vi "Configure Trigger.vi"(8 "error in (no error)":errorcluster, 10 "Params":variant, 11 "ConfigTrigger in":refnum<class "Trigger.lvclass">) -> (0 "error out":errorcluster, 3 "ConfigTrigger out":refnum<class "Trigger.lvclass">)   [LabVIEW 2020, in "Instrument.lvlib" / "Trigger.lvclass"]
uses:
  Trigger.lvclass
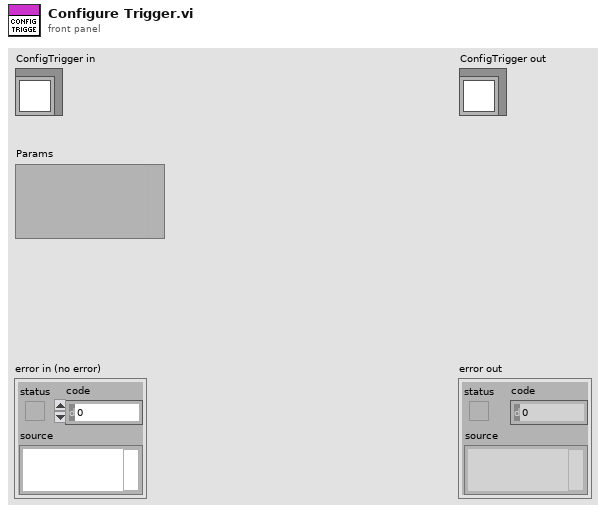
[diagram p1: front panel]
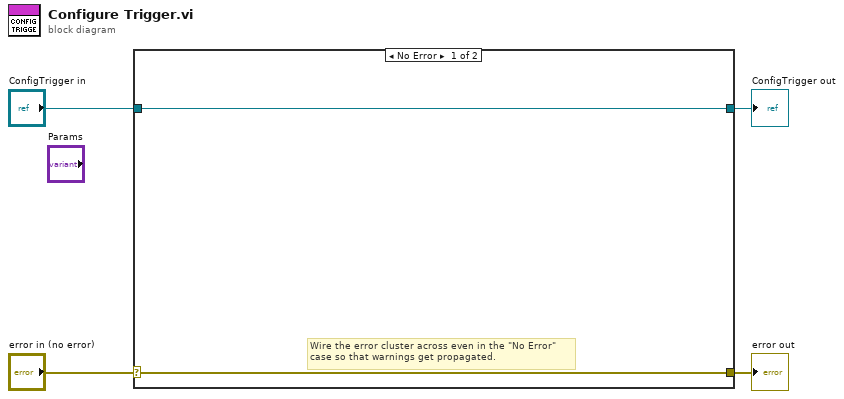
[diagram p0: block diagram]
diagram:
  n1 = case shown="No Error" "error in (no error)" {
    selector: "error in (no error)" -> [w5 w8]
    tunnel: [w5 w8] -> w3
    tunnel: [w6 w7] -> w1
    tunnel: "ConfigTrigger in" -> [w6 w7]
    frame No Error {
      # "Wire the error cluster across even in the \"No Error\"\ncase so that warnings get propagated."
    }
    frame Error {
    }
  }
  "error out" <- w3
  "ConfigTrigger out" <- w1
